vi "Read Spectrum Recorder Configuration.vi"(8 "error in (no error)":errorcluster, 11 "Spectrum Recorder in":refnum<class "Spectrum Recorder too.lvclass">) -> (0 "error out":errorcluster, 2 "Configuration":T1={"Start"=500000.0, "End"=2000000.0, "Duration"=40.0, "Filter time constant"=0.004, "Repeat (-1: forever)"=1, "Update rate"=0.004, "Data storage folder"=path "C:/Data"} {"Update rate" min=0.001 max=10.0 step=0.001 format="%#_6ps"; "Repeat (-1: forever)" format="%.0p"; "Filter time constant" format="%#_6ps"; "Duration" format="%#_6ps"; "End" format="%#_6pHz"; "Start" format="%#_6pHz"}, 3 "Spectrum Recorder out":refnum<class "Spectrum Recorder too.lvclass">)   [LabVIEW 2016, in "Spectrum Recorder too.lvclass"]
uses:
  Spectrum Recorder too.lvclass
  C:/github/Measure_core/Template Module/Template Module.lvclass
  Spectrum Recorder/Spectrum Recorder Configuration.ctl
  Measure_core/Template Module/Template Module.lvclass/Template Module.ctl
  Measure_core/Template Module/Read Configuration.vi
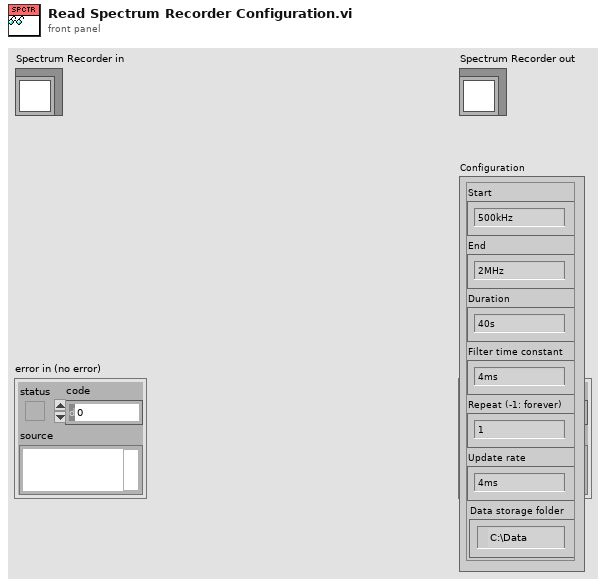
[diagram p1: front panel]
types:
  T1 = typedef "Spectrum Recorder Configuration.ctl" = cluster{"Start":dbl, "End":dbl, "Duration":dbl, "Filter time constant":dbl, "Repeat (-1: forever)":i32, "Update rate":dbl, "Data storage folder":path}
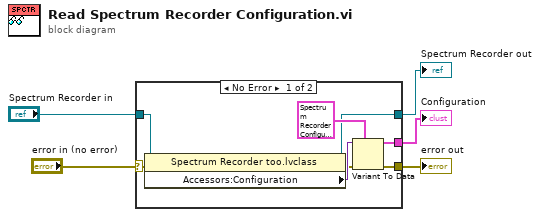
[diagram p0: block diagram]
diagram:
  n1 = case shown="No Error" "error in (no error)" {
    selector: "error in (no error)" -> [w6 w14]
    tunnel: [w10 w14] -> w4
    tunnel: [w9 w15] -> w2
    tunnel: "Spectrum Recorder in" -> [w13 w15]
    tunnel: [w11 _] -> w1
    frame No Error {
      n2 = property class="Spectrum Recorder too.lvclass"(reference=w13, error in=w6) -> (reference out=w9:refnum<class "Spectrum Recorder too.lvclass">, error out=w7:errorcluster, "Accessors:Configuration"=w8:variant)
      n3 = Variant To Data(error in=w7, type=T1 {"Start"=500000.0, "End"=2000000.0, "Duration"=40.0, "Filter time constant"=0.004, "Repeat (-1: forever)"=1, "Update rate"=0.004, "Data storage folder"=path "C:/Data"} ("Configuration"), Variant=w8) -> (data=w11:T1, error out=w10:errorcluster)
    }
    frame Error {
    }
  }
  "error out" <- w4
  "Spectrum Recorder out" <- w2
  "Configuration" <- w1
